vi "Draw_Calculate Height.vi"(8 "Error":errorcluster, 11 "ICON Cluster":T1={"Header"="", "Body"=[], "ImageData"={"image type"=0, "image depth"=0, "image"=[], "mask"=[], "colors"=[], "Rectangle"={"left"=0, "top"=0, "right"=0, "bottom"=0}}, "New Icon"=bytes[0], "Line Status"=[], "Format"={"Color"={"Body txt"=255, "Body Back"=12632256, "Frame"=0, "Header txt"=32768, "Header Back"=16744703, "type"=enum."2 Color"}, "Icon Sizing"={"Rule"=enum."Static", "Header"=TRUE, "Rows"=5, "Width"=32, "Position"=enum."MID-CTR"}}} {"Format"."Icon Sizing"."Rows" min=1 max=5 step=1; "Format"."Icon Sizing"."Width" min=7 max=32 step=1}) -> (0 "Error Out":errorcluster, 3 "Height Out":u32)   [LabVIEW 2009]
uses:
  Controls/Cluster/Cluster_Icon Data.ctl
  Controls/String_Picture/STRING_Line Display.ctl
  Controls/Array/String Array_Body Text.ctl
  Controls/Cluster/Cluster_Image Data.ctl
  Controls/Cluster/CLuster_Selectoin Box.ctl
  Controls/String_Picture/Picture_Icon.ctl
  Controls/Cluster/Cluster_Icon Format.ctl
  Controls/Cluster/Cluster_Icon Color Set.ctl
  Controls/Enum/ENUM_Frame Template Select.ctl
  Controls/Cluster/Cluster_Sizing Data.ctl
  Controls/Enum/ENUM_Icon Sizing.ctl
  Controls/Enum/RBENUM_Icon Position.ctl
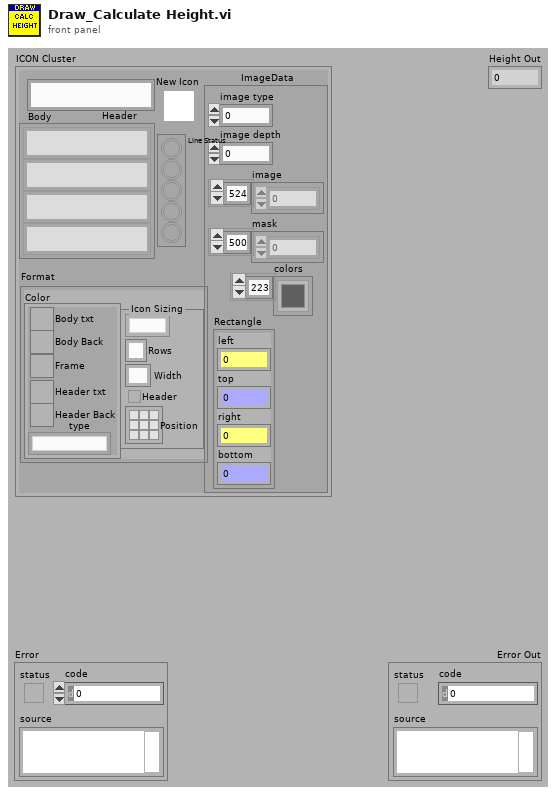
[diagram p1: front panel]
types:
  T1 = typedef "Cluster_Icon Data.ctl" = cluster{"Header":T2, "Body":T3, "ImageData":T4, "New Icon":T6, "Line Status":bool[], "Format":T7}
  T2 = typedef "STRING_Line Display.ctl" = string
  T3 = typedef "String Array_Body Text.ctl" = T2[]
  T4 = typedef "Cluster_Image Data.ctl" = cluster{"image type":i32, "image depth":i32, "image":u8[], "mask":u8[], "colors":u32[], "Rectangle":T5}
  T5 = typedef "CLuster_Selectoin Box.ctl" = cluster{"left":i16, "top":i16, "right":i16, "bottom":i16}
  T6 = typedef "Picture_Icon.ctl" = picture
  T7 = typedef "Cluster_Icon Format.ctl" = cluster{"Color":T8, "Icon Sizing":T10}
  T8 = typedef "Cluster_Icon Color Set.ctl" = cluster{"Body txt":u32, "Body Back":u32, "Frame":u32, "Header txt":u32, "Header Back":u32, "type":T9}
  T9 = typedef "ENUM_Frame Template Select.ctl" = enum16{"2 Color", "5 Color"}
  T10 = typedef "Cluster_Sizing Data.ctl" = cluster{"Rule":T11, "Header":bool, "Rows":u32, "Width":u32, "Position":T12}
  T11 = typedef "ENUM_Icon Sizing.ctl" = enum16{"Static", "Auto"}
  T12 = typedef "RBENUM_Icon Position.ctl" = enum32{"LFT-TOP", "MID-TOP", "RGT-TOP", "LFT-CTR", "MID-CTR", "RGT-CTR", "LFT-BOT", "MID-BOT", "RGT-BOT"}
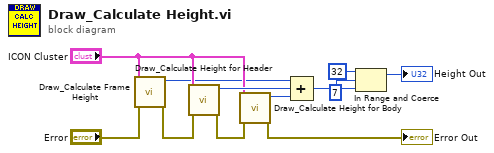
[diagram p0: block diagram]
diagram:
  n1 = call "Draw_Calculate Frame Height.vi"("Error"="Error", "ICON Cluster"="ICON Cluster") -> ("Error Out"=w1:errorcluster, "Height Out"=w3:u32)  [unwired: 8 in]
  n2 = call "Draw_Calculate Height for Header.vi"("Error"=w1, "ICON Cluster"="ICON Cluster") -> ("Error Out"=w8:errorcluster, "Height Out"=w5:u32)  [unwired: 8 in]
  n3 = call "Draw_Calculate Height for Body.vi"("Error"=w8, "ICON Cluster"="ICON Cluster") -> ("Error Out"=→"Error Out":errorcluster, "Height Out"=w6:u32)  [unwired: 8 in]
  n4 = Compound Arithmetic op=ADD(w3, w5, w6) -> (w11:u32)
  n5 = In Range and Coerce(upper limit=u32 32, x=w11, lower limit=u32 7) -> (coerced(x)=→"Height Out":u32)  [unwired: 1 out]
